vi "NMRglobalFM2.vi"() -> ()   [LabVIEW 2013]
uses:
  <vilib>/Analysis/2dsp.llb/Power Spectrum (DBL).vi
  <vilib>/Analysis/NI_AALBase.lvlib
  <vilib>/Analysis/NI_AALPro.lvlib
panel:
  out "FFT Vrms":dbl[](graph)=[0.00491288724422558, 0.004766817799000612, 0.0028347968420014504, 0.00032948259885015016, 0.0007684180461732006, 0.00013461327874688263, 0.0007676915015052642, 0.0003124754799638557, 0.0005542319259414395, 0.0001528235231485258, 0.00012209918011686725, 0.00029999774448873486, 0.00035510982656143626, 0.00012034427911409962, 0.0002622313132652784, 0.00023394631136381392, 0.0004552768836821714, 0.00022947008023570077, 0.00016515382589768265, 0.000533723018673728, 0.00010203360529099216, 0.0001782801878483863, 0.0002684368673757001, 0.0002911776068689857, 2.97512444146063e-05, 0.00025573572949118105, 0.000173696754425059, 0.00021335007604465696, 0.00017095685621183472, 0.0002577887953281745, 7.818504622882473e-05, 0.00023607164482181798, 5.356981939781055e-05, 5.6629280526844514e-05, 8.16922787821161e-05, 0.00013697739713077928, 8.53294702102032e-05, 0.00013239362335425582, 0.00024243690700732426, 0.00033894985716797956, 0.0002711681574789461, 0.0002004623280762697, 0.00018846229233582265, 0.00019547824500197274, 0.0002613330782674258, 0.00017358867498694735, 0.0002622611618019136, 0.00015461352411319805, 2.3075049750455087e-05, 0.00015362372956081617, 0.00018087844752279824, 0.00018087844752279824, 0.00015362372956081617, 2.3075049750455087e-05, 0.00015461352411319805, 0.0002622611618019136, 0.00017358867498694735, 0.0002613330782674258, 0.00019547824500197274, 0.00018846229233582265, 0.0002004623280762697, 0.0002711681574789461, 0.00033894985716797956, 0.00024243690700732426, 0.00013239362335425582, 8.53294702102032e-05, 0.00013697739713077928, 8.16922787821161e-05, 5.6629280526844514e-05, 5.356981939781055e-05, 0.00023607164482181798, 7.818504622882473e-05, 0.0002577887953281745, 0.00017095685621183472, 0.00021335007604465696, 0.000173696754425059, 0.00025573572949118105, 2.97512444146063e-05, 0.0002911776068689857, 0.0002684368673757001, 0.0001782801878483863, 0.00010203360529099216, 0.000533723018673728, 0.00016515382589768265, 0.00022947008023570077, 0.0004552768836821714, 0.00023394631136381392, 0.0002622313132652784, 0.00012034427911409962, 0.00035510982656143626, 0.00029999774448873486, 0.00012209918011686725, 0.0001528235231485258, 0.0005542319259414395, 0.0003124754799638557, 0.0007676915015052642, 0.00013461327874688263, 0.0007684180461732006, 0.00032948259885015016, 0.0028347968420014504, 0.004766817799000612]
  out "NMR Ave Graph":cluster{dbl, "Step Width (MHz)":dbl, dbl[][]}(graph)
  in  "COM Port #":refnum<visa-resource-name>="COM8"
  in  "GPIB Addr (28)":refnum<visa-resource-name>="GPIB0::28::INSTR"
  out "Pedestal (V)":dbl=2.049694229166664 format="%_2g"
  in  "Open Global Panel":bool=TRUE
  out "Peak center (MHz)":sgl=213.36436 format="%.3f"
  out "Telnet error out":errorcluster
  out "+3V supply":dbl=3.294 format="%_4g"
  out "Temp (C)":dbl=28.25 format="%_4g"
  out "RF OK":bool=TRUE
  out "Peak area (V-MHz)":sgl=0.00055034726 format="%.5f"
  out "NMR Graph + Fit":cluster{cluster{dbl, "Numeric":dbl}[]}[](graph)=[{[{213.31, "Numeric"=0.001874778333337268}, {213.311, "Numeric"=0.0018717783333515037}, {213.312, "Numeric"=0.0008088383333650917}, {213.313, "Numeric"=0.006685958333297215}, {213.314, "Numeric"=0.003503138333311284}, {213.315, "Numeric"=0.0002603783333250398}, {213.316, "Numeric"=-0.0030423216666624064}, {213.317, "Numeric"=0.0015950383333502849}, {213.318, "Numeric"=-0.0028275416666381226}, {213.319, "Numeric"=-0.0003100616666973366}, {213.32, "Numeric"=-0.0008525216666850355}, {213.321, "Numeric"=-0.003454921666673272}, {213.322, "Numeric"=-0.004117261666662042}, {213.323, "Numeric"=-0.003839541666651236}, {213.324, "Numeric"=-0.002621761666640854}, {213.325, "Numeric"=-0.004463921666691739}, {213.326, "Numeric"=-0.007366021666681544}, {213.327, "Numeric"=-0.008328061666670994}, {213.328, "Numeric"=-0.007350041666661866}, {213.329, "Numeric"=-0.008431961666652832}, {213.33, "Numeric"=-0.004573821666644662}, {213.331, "Numeric"=-0.004775621666686547}, {213.332, "Numeric"=-0.002037361666678006}, {213.333, "Numeric"=-0.0013590416666695582}, {213.334, "Numeric"=0.0002593383333384658}, {213.335, "Numeric"=0.0008177783333453981}, {213.336, "Numeric"=-0.002683721666647987}, {213.337, "Numeric"=-0.0002451616666823142}, {213.338, "Numeric"=-0.0028665416666751042}, {213.339, "Numeric"=0.003452138333332133}, {213.34, "Numeric"=0.0027108783333380515}, {213.341, "Numeric"=-0.0020903216666563473}, {213.342, "Numeric"=4.853833334861335e-05}, {213.343, "Numeric"=0.0001274583333228385}, {213.344, "Numeric"=0.00014643833332828038}, {213.345, "Numeric"=-0.0008945216666664813}, {213.346, "Numeric"=0.001004578333337669}, {213.347, "Numeric"=0.007843738333341399}, {213.348, "Numeric"=0.0046229583333445845}, {213.349, "Numeric"=0.00834223833332759}, {213.35, "Numeric"=0.011001578333331263}, {213.351, "Numeric"=0.01360097833333418}, {213.352, "Numeric"=0.015140438333337336}, {213.353, "Numeric"=0.009619958333339174}, {213.354, "Numeric"=0.008039538333340701}, {213.355, "Numeric"=0.014399178333332152}, {213.356, "Numeric"=0.018698878333334168}, {213.357, "Numeric"=0.017938638333335533}, {213.358, "Numeric"=0.020118458333336253}, {213.359, "Numeric"=0.015238338333336543}, {213.36, "Numeric"=0.018298278333336526}, {213.361, "Numeric"=0.02129827833333664}, {213.362, "Numeric"=0.020238338333336436}, {213.363, "Numeric"=0.024118458333336257}, {213.364, "Numeric"=0.014938638333335419}, {213.365, "Numeric"=0.02169887833333428}, {213.36599999999999, "Numeric"=0.02039917833333238}, {213.367, "Numeric"=0.020039538333340712}, {213.368, "Numeric"=0.021619958333339184}, {213.369, "Numeric"=0.023140438333337343}, {213.37, "Numeric"=0.019600978333334407}, {213.371, "Numeric"=0.02000157833333116}, {213.37199999999999, "Numeric"=0.015342238333327707}, {213.373, "Numeric"=0.013622958333344481}, {213.374, "Numeric"=0.012843738333341292}, {213.375, "Numeric"=0.01200457833333779}, {213.376, "Numeric"=0.014105478333333643}, {213.377, "Numeric"=0.005146438333328618}, {213.378, "Numeric"=0.004127458333322842}, {213.379, "Numeric"=0.005048538333348507}, {213.38, "Numeric"=0.002909678333343546}, {213.381, "Numeric"=0.006710878333338055}, {213.382, "Numeric"=0.006452138333331803}, {213.383, "Numeric"=0.01313345833332491}, {213.384, "Numeric"=0.007754838333317693}, {213.385, "Numeric"=0.0033162783333522405}, {213.386, "Numeric"=0.004817778333345402}, {213.387, "Numeric"=0.004259338333338469}, {213.388, "Numeric"=0.005640958333330115}, {213.389, "Numeric"=0.0019626383333219977}, {213.39, "Numeric"=-0.0007756216666865434}, {213.391, "Numeric"=-0.0015738216666445481}, {213.392, "Numeric"=-0.0024319616666530486}, {213.393, "Numeric"=-0.0023500416666615287}, {213.394, "Numeric"=-0.0023280616666712106}, {213.395, "Numeric"=-0.002366021666681206}, {213.396, "Numeric"=-0.0014639216666920696}, {213.397, "Numeric"=-0.0006217616666410741}, {213.398, "Numeric"=0.002160458333348547}, {213.399, "Numeric"=-0.00011726166666203852}, {213.4, "Numeric"=0.0015450783333266216}, {213.401, "Numeric"=-0.0018525216666849253}, {213.402, "Numeric"=-0.0013100616666972265}, {213.403, "Numeric"=0.001172458333361881}, {213.404, "Numeric"=0.0015950383333502849}, {213.405, "Numeric"=0.0009576783333375971}, {213.406, "Numeric"=-0.0007396216666748501}, {213.407, "Numeric"=0.0015031383333115045}, {213.408, "Numeric"=0.0036859583332971013}, {213.409, "Numeric"=0.0028088383333653155}, {213.41, "Numeric"=0.0028717783333513935}]}]
  out "# Good Spectra":i32=100
  out "Pedestal OK":bool=TRUE
  out "Sweep #":i32=18
  out "1st Sweep":bool
  out "ADC volts OK":bool=TRUE
  out "Peak Height Distribution":cluster{"Y":dbl[], "Y":dbl[]}[](graph)=[{"Y"=[0.020157212566669552, 0.020308414366669556, 0.02045961616666956, 0.02061081796666956, 0.020762019766669564, 0.020913221566669568, 0.02106442336666957, 0.021215625166669572, 0.021366826966669573, 0.021518028766669577, 0.02166923056666958, 0.02182043236666958, 0.021971634166669585, 0.02212283596666959, 0.02227403776666959, 0.022425239566669593, 0.022576441366669597, 0.022727643166669597, 0.0228788449666696, 0.0230300467666696, 0.023181248566669605, 0.02333245036666961, 0.02348365216666961, 0.023634853966669613, 0.023786055766669617, 0.023937257566669617, 0.02408845936666962, 0.024239661166669625, 0.024390862966669626, 0.02454206476666963, 0.024693266566669633, 0.024844468366669634, 0.024995670166669638, 0.025146871966669638, 0.025298073766669642, 0.025449275566669646, 0.025600477366669646, 0.02575167916666965, 0.025902880966669654, 0.026054082766669654, 0.026205284566669658, 0.026356486366669662, 0.026507688166669662, 0.026658889966669666, 0.026810091766669666, 0.02696129356666967, 0.027112495366669674, 0.027263697166669675, 0.02741489896666968, 0.027566100766669682, 0.027717302566669683, 0.027868504366669686, 0.02801970616666969, 0.02817090796666969, 0.028322109766669695, 0.0284733115666697, 0.0286245133666697, 0.028775715166669703, 0.028926916966669703, 0.029078118766669707, 0.02922932056666971, 0.02938052236666971, 0.029531724166669715, 0.02968292596666972, 0.02983412776666972, 0.029985329566669723, 0.030136531366669727, 0.030287733166669727, 0.03043893496666973, 0.03059013676666973, 0.030741338566669735, 0.03089254036666974, 0.03104374216666974, 0.031194943966669744, 0.03134614576666975, 0.03149734756666975, 0.03164854936666975, 0.031799751166669755, 0.031950952966669756, 0.032102154766669756, 0.032253356566669764, 0.032404558366669764, 0.032555760166669764, 0.03270696196666977, 0.03285816376666977, 0.03300936556666977, 0.03316056736666978, 0.03331176916666978, 0.03346297096666978, 0.03361417276666979, 0.03376537456666979, 0.03391657636666979, 0.034067778166669796, 0.034218979966669796, 0.0343701817666698, 0.034521383566669804, 0.034672585366669804, 0.034823787166669805, 0.03497498896666981, 0.03512619076666981], "Y"=[1.0, 0.0, 0.0, 1.0, 0.0, 0.0, 1.0, 0.0, 0.0, 1.0, 0.0, 0.0, 2.0, 0.0, 2.0, 0.0, 0.0, 0.0, 0.0, 0.0, 1.0, 2.0, 2.0, 1.0, 3.0, 1.0, 1.0, 1.0, 2.0, 0.0, 0.0, 0.0, 0.0, 0.0, 3.0, 1.0, 2.0, 3.0, 2.0, 1.0, 4.0, 1.0, 2.0, 2.0, 0.0, 1.0, 3.0, 0.0, 4.0, 2.0, 2.0, 0.0, 1.0, 7.0, 5.0, 2.0, 1.0, 0.0, 2.0, 3.0, 1.0, 1.0, 3.0, 1.0, 2.0, 0.0, 2.0, 2.0, 1.0, 0.0, 1.0, 0.0, 2.0, 0.0, 1.0, 0.0, 1.0, 0.0, 1.0, 0.0, 0.0, 0.0, 0.0, 0.0, 0.0, 0.0, 1.0, 0.0, 0.0, 2.0, 0.0, 0.0, 1.0, 0.0, 0.0, 0.0, 0.0, 0.0, 0.0, 1.0]}]
  out "S/N":dbl=8.889914894885075 format="%_3g"
  out "Peak mean (V)":dbl=0.027208529933335814 format="%_4g"
  out "Pedestal Diff (V)":sgl=0.00362787 format="%.3f"
  out "Peak amp (V)":sgl=0.024118459 format="%.3f"
  out "SMT error out":errorcluster
  out "Sample RMS (V)":dbl format="%.4f"
  # "E1039 NMR Panel"
  # "Results"
  # "A\nv\ne\nr\na\ng\ne"
  # "S\nw\ne\ne\np"
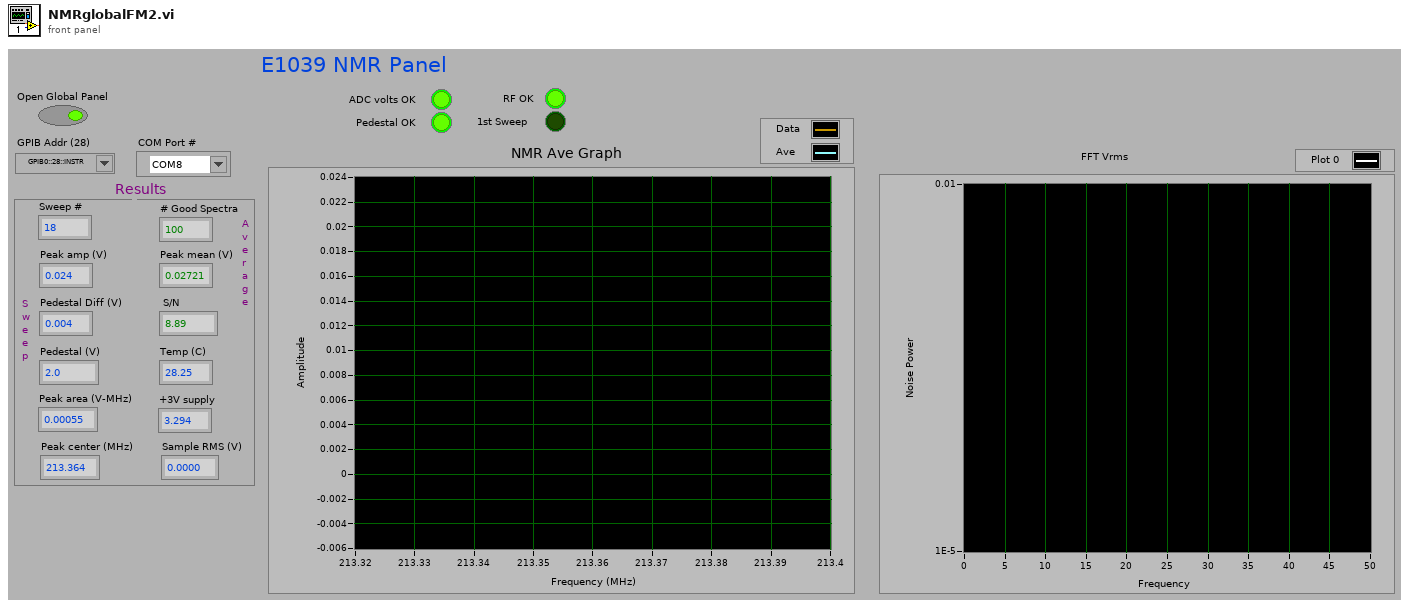
[diagram p1: front panel]
types:
  T1 = enum32{"Invalid", "Standard", "Closed", "Hidden", "Minimized", "Maximized"}
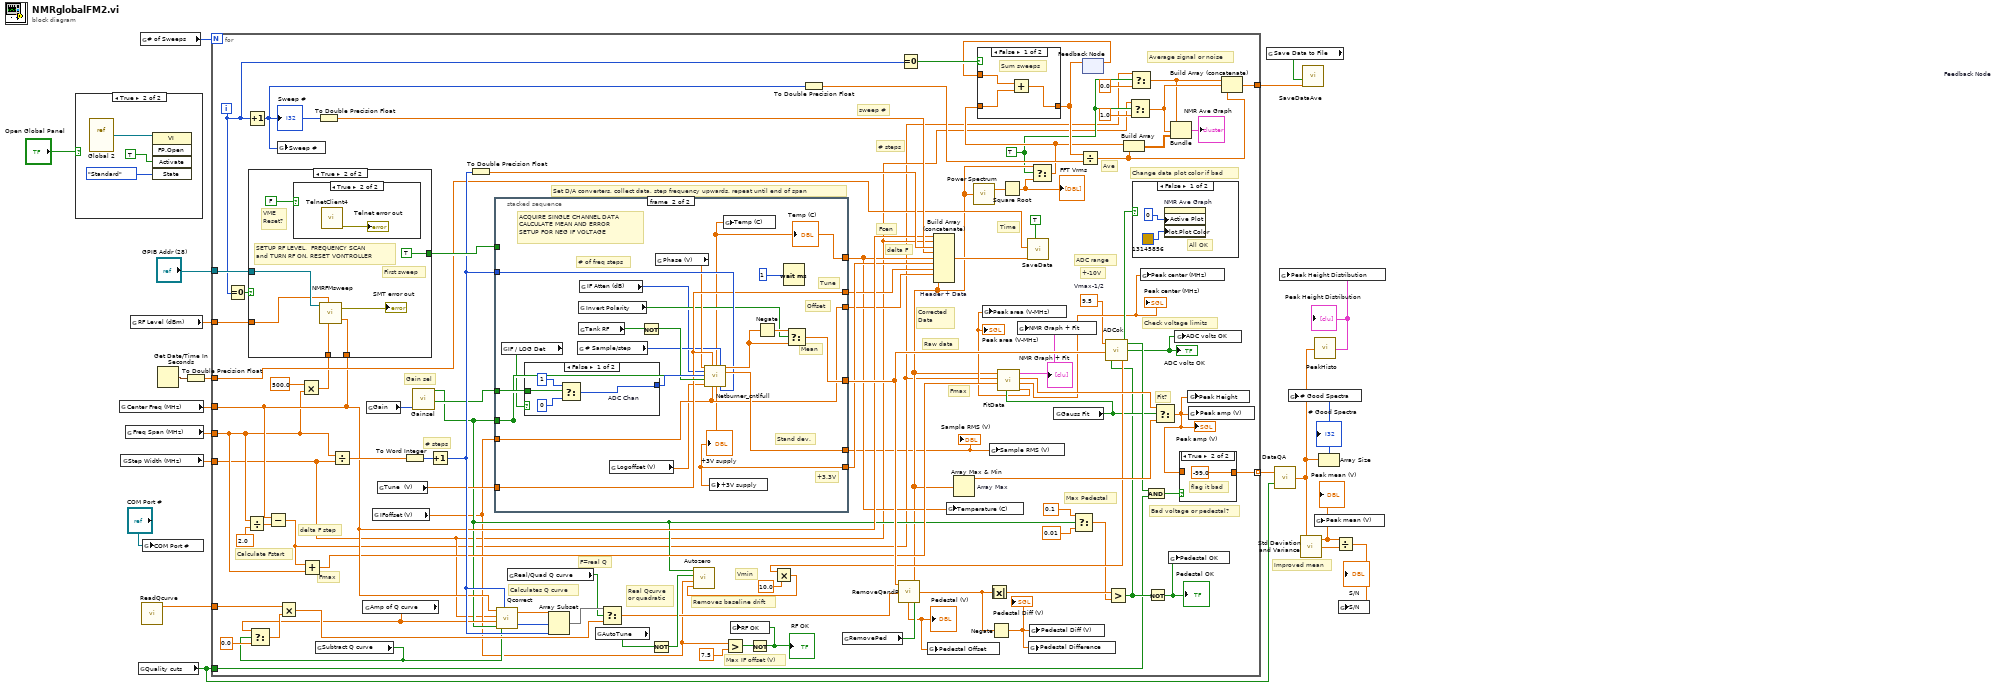
[diagram p0: block diagram]
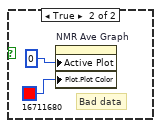
[diagram p4: hidden frame]
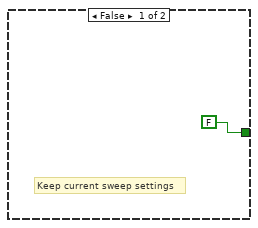
[diagram p6: hidden frame]
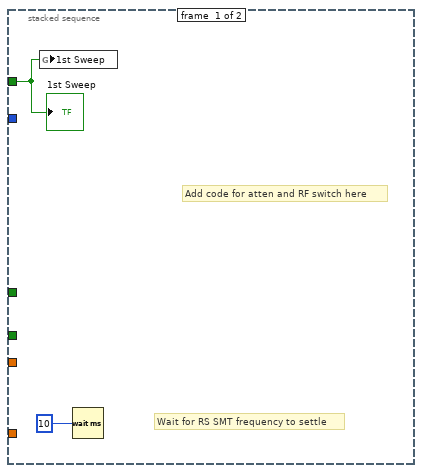
[diagram p8: hidden frame]
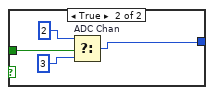
[diagram p9: hidden frame]
diagram:
  # "Improved mean"
  n1 = case shown="True" "Open Global Panel" {
    frame False {
    }
    frame True {
      n2 = vi-ref "Global 2.vi"() -> (w24:refnum<vi>)
      n3 = invoke class="VI" method="FP.Open"(reference=w24, "Activate"=TRUE, "State"=T1."Standard") -> ()  [unwired: 2 in, 5 out]
    }
  }
  n4 = global read "Global 2.vi" "Center Freq (MHz)"() -> (w15:dbl)
  n5 = global read "Global 2.vi" "Step Width (MHz)"() -> (w13:dbl)
  n6 = global read "Global 2.vi" "Freq Span (MHz)"() -> (w14:dbl)
  n7 = global read "Global 2.vi" "RF Level (dBm)"() -> (w16:dbl)
  n8 = global read "Global 2.vi" "Quality cuts"() -> (w12:bool)
  n9 = global read "Global 2.vi" "# of Sweeps"() -> (w17:i32)
  n10 = call "ReadQcurve.vi"() -> ("Array"=w1:dbl[])  [unwired: 2 in]
  n11 = global write "Global 2.vi" "COM Port #"("COM Port #") -> ()
  n12 = Get Date/Time In Seconds() -> (seconds since 1Jan1904=w19:timestamp)
  n13 = To Double Precision Float(number=w19) -> (double precision float=w2:dbl)
  n14 = for {
    N: w17 -> [_]
    tunnel: [w109] -> w21 mode=indexing
    tunnel: w12 -> [w58]
    tunnel: w15 -> [w95]
    tunnel: w14 -> [w38]
    tunnel: w13 -> [w28]
    tunnel: "GPIB Addr (28)" -> [w102]
    tunnel: w16 -> [w101]
    tunnel: w2 -> [w99]
    tunnel: w1 -> [w88]
    tunnel: [w44] -> w4
    i -> [w40]
    w30 = TRUE
    w52 = 9.5  # Vmax-1/2
    # "Average signal or noise"
    # "Check voltage limits"
    # "Ave"
    # "Max Pedestal"
    # "Gain sel"
    # "F=real Q"
    # "Real Qcurve\nor quadratic"
    # "+-10V"
    # "Change data plot color if bad"
    # "Max IF offset (V)"
    # "Fmax"
    # "Fit?"
    # "Fmax"
    # "Time"
    # "Vmin"
    # "Raw data"
    # "Corrected\nData"
    # "Fcen"
    # "delta F"
    # "# steps"
    # "ADC range"
    # "sweep #"
    # "Set D/A converters, collect data, step frequency upwards, repeat until end of span"
    # "Calculates Q curve"
    # "Removes baseline drift"
    # "Bad voltage or pedestal?"
    # "# steps"
    # "Calculate Fstart"
    # "delta F step"
    n15 = Equal To 0?(x=w40) -> (x = 0?=w111:bool)
    n16 = Divide(x=w38, y=sgl 2.0) -> (x/y=w115:dbl)
    n17 = Increment(x=w40) -> (x+1=w56:i32)
    "Sweep #" <- w56
    n18 = Subtract(x=w95, y=w115) -> (x-y=w27:dbl)
    n19 = global write "Global 2.vi" "Sweep #"(w56) -> ()
    n20 = Multiply(x=500.0, y=w38) -> (x*y=w37:dbl)
    n21 = case shown="True" w111 {
      tunnel: w95 -> [_ w134]
      tunnel: w37 -> [_ w135]
      tunnel: [FALSE TRUE] -> w110
      tunnel: w102 -> [_ w131]
      tunnel: w101 -> [_ w130]
      frame False {
        # "Keep current sweep settings"
      }
      frame True {
        # "VME\nReset?"
        # "First sweep"
        # "SETUP RF LEVEL,  FREQUENCY SCAN\nand TURN RF ON. RESET VONTROLLER"
        n22 = case shown="True" FALSE {
          frame False {
          }
          frame True {
            n23 = call "TelnetClient4.vi"() -> ("Telnet error"=→"Telnet error out":errorcluster)  [unwired: 4 in, 3 out]
          }
        }
        n24 = call "NMRFMsweep.vi"("Center Freq (MHz)"=w134, "Freq Span (kHz)"=w135, "RF Level (dBm)"=w130, "GPIB Addr (28)"=w131) -> ("error out"=→"SMT error out":errorcluster)  [unwired: 3 in]
      }
    }
    n25 = Add(x=w27, y=w38) -> (x+y=w93:dbl)
    n26 = global read "Global 2.vi" "Subtract Q curve"() -> (w76:bool)
    n27 = To Double Precision Float(number=w56) -> (double precision float=w103:dbl)
    n28 = Divide(x=w38, y=w28) -> (x/y=w117:dbl)
    n29 = global read "Global 2.vi" "Amp of Q curve"() -> (w77:dbl)
    n30 = Select(t=w77, s=w76, f=0.0) -> (s? t:f=w85:dbl)
    n31 = Multiply(x=w88, y=w85) -> (x*y=w87:dbl[])
    n32 = global read "Global 2.vi" "Gain"() -> (w47:enum16{"LOW", "HI", "MAX"})
    n33 = global read "Global 2.vi" "IFoffset (V)"() -> (w43:dbl)
    n34 = global read "Global 2.vi" "Tune  (V)"() -> (w78:dbl)
    n35 = To Word Integer(number=w117) -> (16bit integer=w114:i16)
    n36 = call "Gainsel.vi"("Gain"=w47) -> ("LO"=w48:bool, "MAX"=w46:bool)  [unwired: 1 out]
    n37 = Increment(x=w114) -> (x+1=w105:i16)
    n38 = To Double Precision Float(number=w105) -> (double precision float=w104:dbl)
    n39 = stacked-sequence {
      tunnel: [_ w154] -> w25
      tunnel: [_ w158] -> w100
      tunnel: w105 -> [_ w152]
      tunnel: w43 -> [_ w149]
      tunnel: w48 -> [_ w156]
      tunnel: w110 -> [w137 _]
      tunnel: w78 -> [_ w150]
      tunnel: [_ w140] -> w63
      tunnel: [_ w139] -> w84
      tunnel: [_ w150] -> w83
      tunnel: [_ w149] -> w82
      tunnel: [_ w148] -> _
      tunnel: w46 -> [_ w148]
      frame #0 {
        # "Add code for atten and RF switch here"
        # "Wait for RS SMT frequency to settle"
        n40 = global write "Global 2.vi" "1st Sweep"(w137) -> ()
        n41 = Wait (ms)(milliseconds to wait=10) -> ()  [unwired: 1 out]
        "1st Sweep" <- w137
      }
      frame #1 {
        # "+3.3V"
        # "Offset"
        # "Tune"
        # "Stand dev."
        # "Mean"
        # "ACQUIRE SINGLE CHANNEL DATA\nCALCULATE MEAN AND ERROR\nSETUP FOR NEG IF VOLTAGE"
        # "# of freq steps"
        n42 = global read "Global 2.vi" "IF / LOG Det"() -> (w145:bool)
        n43 = case shown="False" w145 {
          tunnel: w156 -> [w163 w164]
          tunnel: [w160 w165] -> w153
          frame False {
            n44 = Select "ADC Chan"(t=1, s=w163, f=0) -> (s? t:f=w160:i32)
          }
          frame True {
            n45 = Select "ADC Chan"(t=2, s=w164, f=3) -> (s? t:f=w165:i32)
          }
        }
        n46 = global read "Global 2.vi" "# Sample/step"() -> (w142:i32)
        n47 = global read "Global 2.vi" "Tank RF"() -> (w144:bool)
        n48 = global read "Global 2.vi" "Invert Polarity"() -> (w143:bool)
        n49 = global read "Global 2.vi" "IF Atten (dB)"() -> (w141:i8)
        n50 = global read "Global 2.vi" "Logoffset (V)"() -> (w146:dbl)
        n51 = Not(x=w144) -> (.not. x?=w151:bool)
        n52 = global read "Global 2.vi" "Phase (V)"() -> (w147:dbl)
        n53 = call "Netburner_cntlfull.vi"("Phase Volt"=w147, "Tune Volt"=w150, "# Data"=w142, "IF Atten (dB)"=w141, "NMR ADC"=w153, "Hi Gain"=w148, "Tank RF"=w151, "LogOff Volt"=w146, "IFOff Volt"=w149, "# f steps"=w152) -> ("Temp (C)"=w140:dbl, "ADC value"=w155:dbl[], "ADC Std Dev"=w154:dbl, "Volts"=w139:dbl)  [unwired: 2 out]
        "Temp (C)" <- w140
        "+3V supply" <- w139
        n54 = global write "Global 2.vi" "+3V supply"(w139) -> ()
        n55 = global write "Global 2.vi" "Temp (C)"(w140) -> ()
        n56 = Negate(x=w155) -> (-x=w157:dbl[])
        n57 = Wait (ms)(milliseconds to wait=1) -> ()  [unwired: 1 out]
        n58 = Select(t=w157, s=w143, f=w155) -> (s? t:f=w158:dbl[])
      }
    }
    "Sample RMS (V)" <- w25
    n59 = call "Qcorrect.vi"("Subtract Q curve"=w76, "Nstep"=w105, "Max Gain"=w46, "Amp of Q curve"=w77, "Step Width (MHz)"=w28, "Center Freq (MHz)"=w95) -> ("Start"=w112:i32, "Array"=w113:dbl[])
    n60 = global read "Global 2.vi" "Real/Quad Q curve"() -> (w75:bool)
    n61 = Array Subset "Array Subset"(array=w113, index=w112, length=w105) -> (w90:dbl[])
    n62 = global read "Global 2.vi" "AutoTune"() -> (w73:bool)
    n63 = Select(t=w90, s=w75, f=w87) -> (s? t:f=w89:dbl[])
    n64 = Not(x=w73) -> (.not. x?=w91:bool)
    n65 = Greater?(x=w43, y=7.5) -> (0:w96:bool)
    n66 = Not(x=w96) -> (.not. x?=w69:bool)
    "RF OK" <- w69
    n67 = global write "Global 2.vi" "RF OK"(w69) -> ()
    n68 = To Double Precision Float(number=w56) -> (double precision float=w50:dbl)
    n69 = global read "Global 2.vi" "RemovePed"() -> (w74:bool)
    n70 = call "RemoveQandP.vi"("Subtract Ped?"=w74, "Qcurve"=w89, "Raw data"=w100) -> ("Ped L-R"=w106:dbl, "Corrected data"=w34:dbl[], "Ped Offfset"=w62:dbl)
    "Pedestal (V)" <- w62
    n71 = Equal To 0?(x=w40) -> (x = 0?=w55:bool)
    n72 = global write "Global 2.vi" "Pedestal Offset"(w62) -> ()
    n73 = Build Array (concatenate) "Header + Data"(w95, w28, w104, w103, w63, w84, w83, w82, w34) -> (w41:dbl[])
    n74 = global write "Global 2.vi" "Temperature (C)"(w63) -> ()
    n75 = Array Max & Min "Array Max"(array=w34) -> (max value=w98:dbl)  [unwired: 3 out]
    n76 = call-poly <vilib>:"Power Spectrum.vi"("X"=w34) -> ("Power Spectrum"=w39:dbl[])  [unwired: 1 out]
    n77 = Absolute Value ("Abs Value")(x=w106) -> (abs(x)=w107:dbl)
    n78 = global write "Global 2.vi" "Sample RMS (V)"(w25) -> ()
    n79 = Negate(x=w106) -> (-x=w64:dbl)
    "Pedestal Diff (V)" <- w64
    n80 = Square Root(x=w39) -> (sqrt(x)=w35:dbl[])
    "FFT Vrms" <- w35
    n81 = call "SaveData.vi"("Array"=w41, "Save Data to File"=TRUE, "Ext time (sec)"=w99) -> ()  [unwired: 1 out]
    n82 = global write "Global 2.vi" "Pedestal Difference"(w64) -> ()
    n83 = global write "Global 2.vi" "Pedestal Diff (V)"(w64) -> ()
    n84 = Select(t=w34, s=w30, f=w35) -> (s? t:f=w33:dbl[])
    n85 = global read "Global 2.vi" "Gauss Fit"() -> (w72:bool)
    n86 = call "FitData.vi"("Fit?"=w72, "Fmax"=w93, "Fmin"=w27, "Yarray"=w34) -> ("Peak Area (V-MHz)"=w68:dbl, "Center Freq (MHz)"=w67:dbl, "Amplitude (V)"=w94:dbl, "NMR Graph + Fit"=w65:cluster{cluster{dbl, "Numeric":dbl}[]}[])  [unwired: 1 out]
    "NMR Graph + Fit" <- w65
    "Peak area (V-MHz)" <- w68
    "Peak center (MHz)" <- w67
    n87 = global write "Global 2.vi" "Peak area (V-MHz)"(w68) -> ()
    n88 = global write "Global 2.vi" "NMR Graph + Fit"(w65) -> ()
    n89 = Select(t=0.1, s=w46, f=0.01) -> (s? t:f=w57:dbl)
    n90 = feedback #1 "Feedback Node"() -> (w54:dbl[])  [unwired: 1 in]
    n91 = case shown="False" w55 {
      tunnel: w33 -> [w119 w121]
      tunnel: [w118 w121] -> w51
      tunnel: w54 -> [w120 _]
      frame False {
        # "Sum sweeps"
        n92 = Add(x=w120, y=w119) -> (x+y=w118:dbl[])
      }
      frame True {
        # "Initialize"
      }
    }
    n93 = Divide(x=w51, y=w50) -> (x/y=w45:dbl[])
    n94 = feedback-in #1(w51) -> ()
    n95 = Greater?(x=w107, y=w57) -> (0:w59:bool)
    n96 = call "ADCok.vi"("PedOK"=w59, "Array"=w100, "Vmax-1/2"=w52) -> ("Vmin"=w81:dbl, "ADC voltages OK"=w71:bool, "Allok"=w92:bool)
    "ADC volts OK" <- w71
    n97 = Multiply(x=w81, y=10.0) -> (x*y=w79:dbl)
    n98 = call "Autozero.vi"("Vmin (V)"=w79, "IFoffset (V)"=w43, "Enable"=w91, "Max Gain"=w46) -> ()
    n99 = Build Array "Build Array"(w33, w45) -> (w49:dbl[][])
    n100 = Select(t=w28, s=w30, f=1.0) -> (s? t:f=w31:dbl)
    n101 = Select(t=w27, s=w30, f=0.0) -> (s? t:f=w26:dbl)
    n102 = case shown="False" w92 {
      frame False {
        # "All OK"
        n103 = property on="NMR Ave Graph" class="WFGraph (strict)"("Active Plot"=0, "Plot.Plot Color"=u32 13145856) -> ()  [unwired: 2 in, 2 out]
      }
      frame True {
        # "Bad data"
        n104 = property on="NMR Ave Graph" class="WFGraph (strict)"("Active Plot"=0, "Plot.Plot Color"=u32 16711680) -> ()  [unwired: 2 in, 2 out]
      }
    }
    n105 = global write "Global 2.vi" "Peak center (MHz)"(w67) -> ()
    n106 = And(x=w92, y=w58) -> (x .and. y?=w108:bool)
    n107 = Not(x=w59) -> (.not. x?=w70:bool)
    "Pedestal OK" <- w70
    n108 = Select(t=w94, s=w72, f=w98) -> (s? t:f=w66:dbl)
    "Peak amp (V)" <- w66
    n109 = global write "Global 2.vi" "Pedestal OK"(w70) -> ()
    n110 = Bundle(w26, "Step Width (MHz)"=w31, w49) -> (→"NMR Ave Graph":cluster{dbl, "Step Width (MHz)":dbl, dbl[][]})  [unwired: 1 in]
    n111 = global write "Global 2.vi" "ADC volts OK"(w71) -> ()
    n112 = case shown="True" w108 {
      tunnel: [w126 -99.0] -> w109
      tunnel: w66 -> [w126 _]
      frame False {
        # "Data OK"
      }
      frame True {
        # "flag it bad"
      }
    }
    n113 = global write "Global 2.vi" "Peak Height"(w66) -> ()
    n114 = global write "Global 2.vi" "Peak amp (V)"(w66) -> ()
    n115 = Build Array (concatenate) "Build Array"(w26, w31, w45) -> (w44:dbl[])
  }
  n116 = global read "Global 2.vi" "Save Data to File"() -> (w3:bool)
  n117 = call "DataQA.vi"("Quality cuts"=w12, "Data In"=w21) -> ("Data Out"=w20:dbl[])
  n118 = call <vilib>:"Std Deviation and Variance.vi"("X"=w20) -> ("mean"=w10:dbl, "standard deviation"=w18:dbl)  [unwired: 1 in, 1 out]
  "Peak mean (V)" <- w10
  n119 = call "SaveDataAve.vi"("Array"=w4, "Save Data to File"=w3) -> ()  [unwired: 1 in, 1 out]
  n120 = call "PeakHisto.vi"("Data Out"=w20) -> ("XY Graph"=w8:cluster{"Y":dbl[], "Y":dbl[]}[])
  "Peak Height Distribution" <- w8
  n121 = global write "Global 2.vi" "Peak Height Distribution"(w8) -> ()
  n122 = global write "Global 2.vi" "Peak mean (V)"(w10) -> ()
  n123 = Array Size(array=w20) -> (size(s)=w9:i32)
  "# Good Spectra" <- w9
  n124 = global write "Global 2.vi" "# Good Spectra"(w9) -> ()
  n125 = Divide(x=w10, y=w18) -> (x/y=w11:dbl)
  "S/N" <- w11
  n126 = global write "Global 2.vi" "S/N"(w11) -> ()
